vi "HTS Front Panel.vi"() -> ()   [LabVIEW 2019, in "Results.lvlib" / "HTS Results.lvclass"]
uses:
  HTS Results.lvclass
  HTS Results.lvclass/HTS Results.ctl
  Test Stands/HTS/HTS Test Stand.lvclass
panel:
  out "HTS dU":dbl caption="HTS dU, uV" format="%#.1f"
  out "LN2 Temp":dbl caption="LN2 Temp, K" format="%#.2f"
  in  "Supp U ctrl":dbl caption="Supp U ctrl, V"
  in  "Supp I ctrl":dbl caption="Supp I ctrl, A"
  out "Supp U":dbl caption="Supp U, V" format="%#.3f"
  out "Supp I":dbl caption="Supp I, A" format="%#.2f"
  out "Absolute Pressure, bar":dbl(knob)=1.0 scale=0.0..1.0
  out "Vac Pressure, bar(a)":dbl=1.0 format="%#.5f"
  out "Vac Press I":dbl caption="Vac Press I, mA" format="%#.3f"
  out "Valve Position":dbl caption="Vacuum Valve Position, % open"
  in  "Valve Position":dbl caption="Vacuum Valve Position, % open" min=0.0 max=100.0 step=1.0
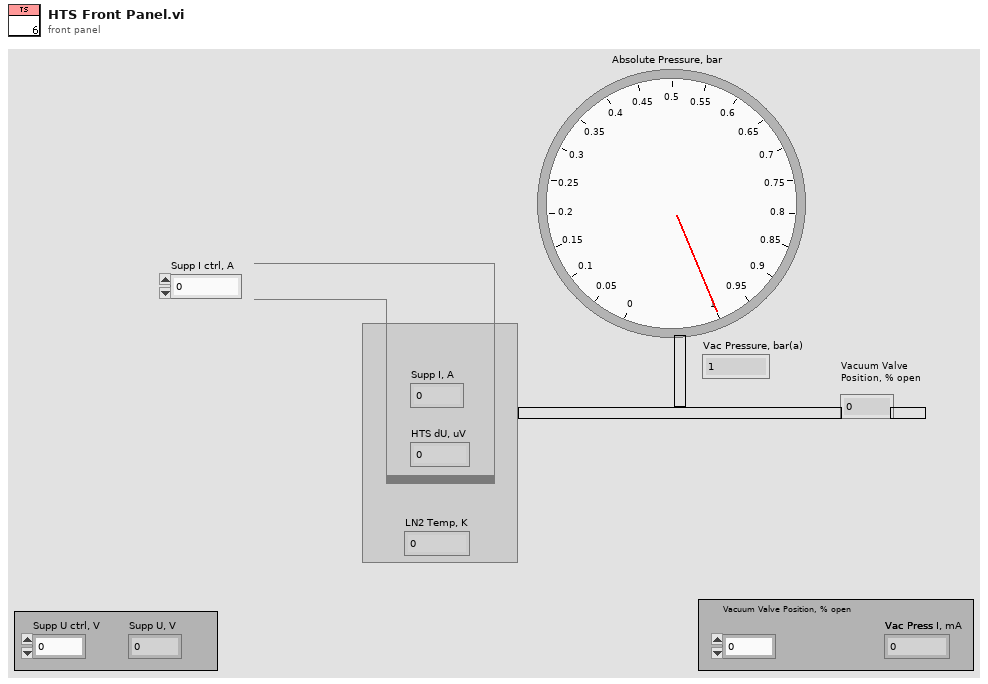
[diagram p1: front panel]
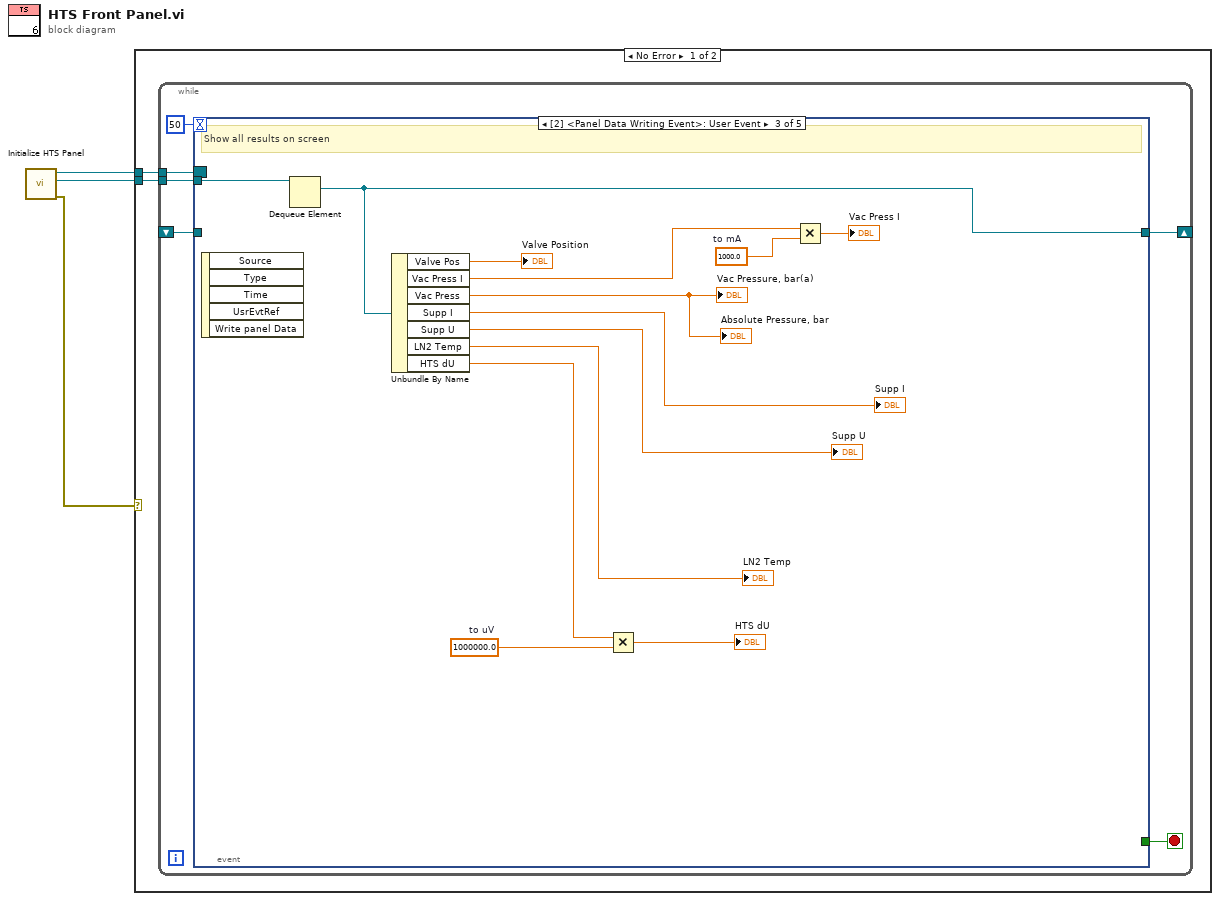
[diagram p0: block diagram]
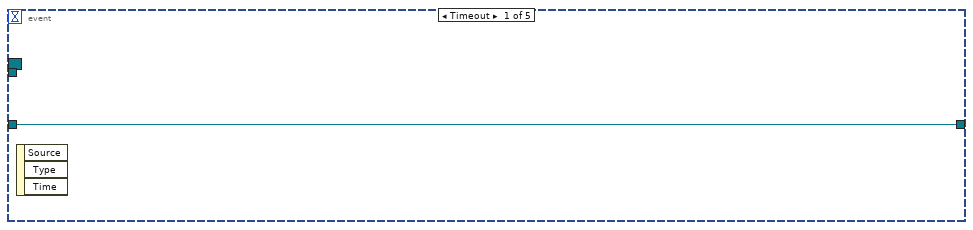
[diagram p2: hidden frame]
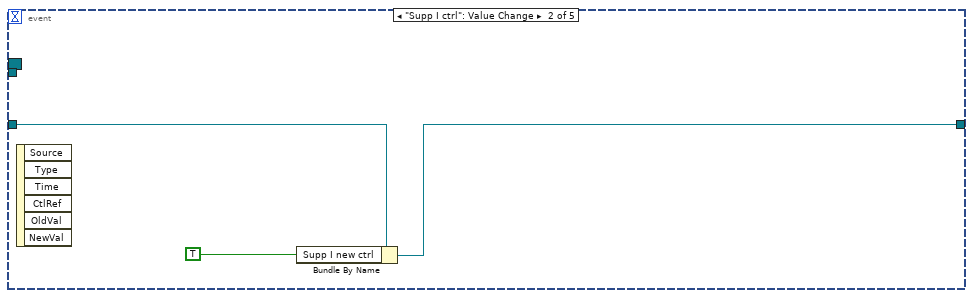
[diagram p3: hidden frame]
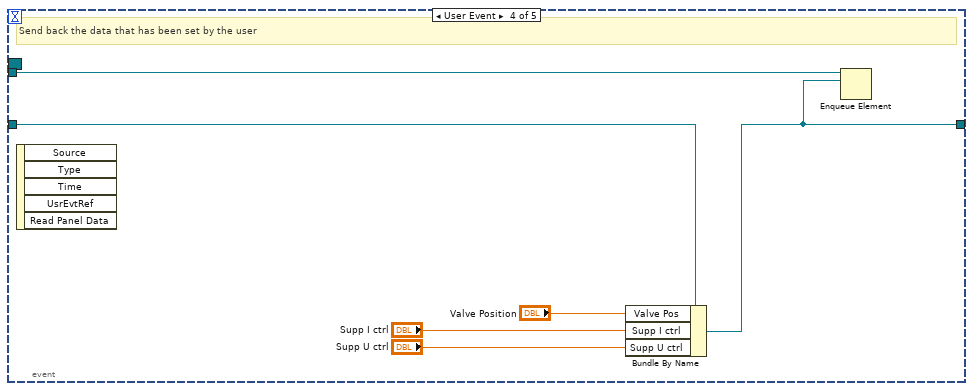
[diagram p4: hidden frame]
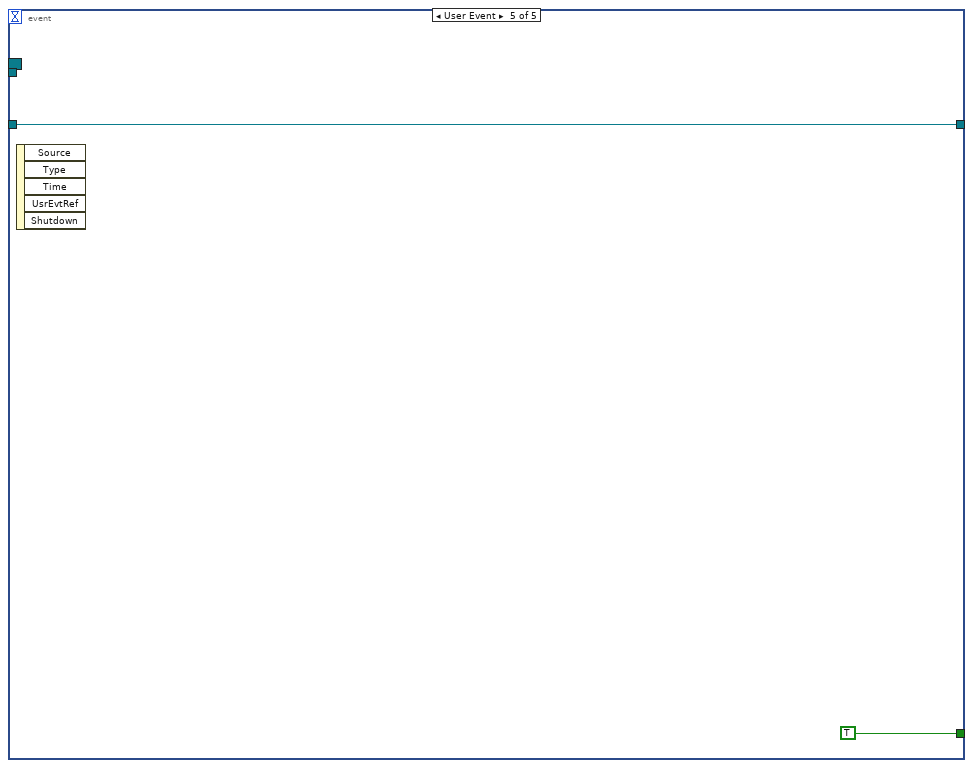
[diagram p5: hidden frame]
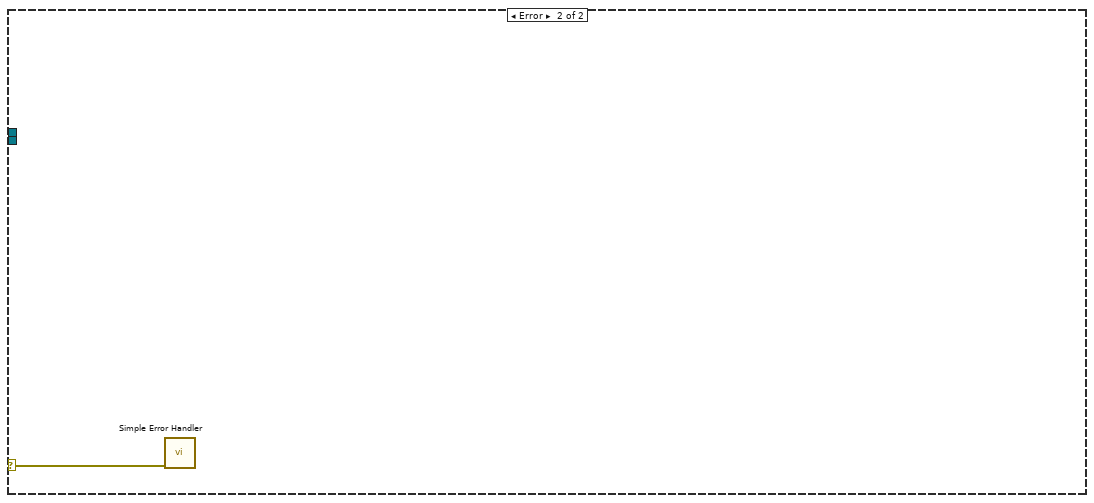
[diagram p6: hidden frame]
diagram:
  n1 = call "Initialize HTS Panel.vi"() -> ("error out"=w2:errorcluster, "HTS Results queue out"=w1:refnum<queue>, "Event Registration Refnum"=w3:refnum<event-registration>)  [unwired: 9 in]
  n2 = case shown="No Error" w2 {
    selector: w2 -> [_ w37]
    tunnel: w3 -> [w5 _]
    tunnel: w1 -> [w4 _]
    frame No Error {
      n3 = while {
        tunnel: w5 -> [w10]
        tunnel: w4 -> [w9]
        shift-right: [w7] -> _
        shift-left: _ -> [w6]
        stop <- w11 stop-if-true
        n4 = event shown="[2] <Panel Data Writing Event>: User Event" {
          selector: w10 -> [_ _ _ _ _]
          dyn-events: _ -> [_ _ _ _ _]
          timeout: 50 -> [_ _ _ _ _]
          tunnel: [_ _ _ _ TRUE] -> w11
          tunnel: w9 -> [_ _ w28 w34 _]
          tunnel: [w12 w14 w27 w32 w35] -> w7
          tunnel: w6 -> [w12 w15 _ w33 w35]
          event Timeout {
            n5 = event-data() -> ()  [unwired: 1 in, 3 out]
          }
          event "Supp I ctrl": Value Change {
            n6 = event-data() -> ()  [unwired: 1 in, 6 out]
            n7 = Bundle By Name(cluster=w15, "Supp I new ctrl"=TRUE) -> (w14:refnum<class "HTS Results.lvclass">)
          }
          event User Event {
            w17 = 1000.0  # to mA
            w20 = 1000000.0  # to uV
            # "Show all results on screen"
            n8 = event-data() -> ()  [unwired: 1 in, 5 out]
            n9 = Dequeue Element(queue=w28) -> (element=w27:refnum<class "HTS Results.lvclass">)  [unwired: 2 in, 3 out]
            n10 = Unbundle By Name(w27) -> ("Valve Pos"=→"Valve Position":dbl, "Vac Press I"=w18:dbl, "Vac Press"=→"Vac Pressure, bar(a)" →"Absolute Pressure, bar":dbl, "Supp I"=→"Supp I":dbl, "Supp U"=→"Supp U":dbl, "LN2 Temp"=→"LN2 Temp":dbl, "HTS dU"=w21:dbl)
            n11 = Multiply(x=w21, y=w20) -> (x*y=→"HTS dU":dbl)
            n12 = Multiply(x=w18, y=w17) -> (x*y=→"Vac Press I":dbl)
          }
          event User Event {
            # "Send back the data that has been set by the user"
            n13 = event-data() -> ()  [unwired: 1 in, 5 out]
            n14 = Bundle By Name(cluster=w33, "Valve Pos"="Valve Position", "Supp I ctrl"="Supp I ctrl", "Supp U ctrl"="Supp U ctrl") -> (w32:refnum<class "HTS Results.lvclass">)
            n15 = Enqueue Element(queue=w34, element=w32) -> ()  [unwired: 2 in, 3 out]
          }
          event User Event {
            n16 = event-data() -> ()  [unwired: 1 in, 5 out]
          }
        }
      }
    }
    frame Error {
      n17 = call <vilib>:"Simple Error Handler.vi"("error in (no error)"=w37) -> ()  [unwired: 4 in, 5 out]
    }
  }
